vi "Mutation Frame.vi"(8 "error in (no error)":errorcluster, 10 "OSSP_Problem":refnum<class "OSSP_Problem.lvclass">, 11 "GA in":refnum<class "GA.lvclass">) -> (0 "error out":errorcluster, 2 "OSSP_Problem Out":refnum<class "OSSP_Problem.lvclass">, 3 "GA out":refnum<class "GA.lvclass">)   [LabVIEW 2013, in "GA.lvclass"]
uses:
  GA.lvclass
  OSSP_Problem.lvclass
  GA.lvclass/GA.ctl
  SA_Class/Controls/Perturbation Method.ctl
  OSSP_Problem.lvclass/OSSP_Problem.ctl
  SA.lvclass/SA.ctl
  SA_Class/Setters/Write Alpha Value.vi
  SA_Class/Setters/Write Current Temperature.vi
  SA_Class/Setters/Write Cooling Strategy.vi
  SA_Class/Setters/Write Initial Temperature.vi
  SA_Class/Setters/Write Stop Temperature.vi
  SA_Class/Setters/Write Cooling Rate.vi
  SA_Class/Setters/Write Epoch Length.vi
  SA_Class/Setters/Write Current Solution.vi
  SA_Class/Setters/Write Best Solution.vi
  GA/SubVIS/Calcualte General Tardiness.vi
  Scheduler_Class/Giffler Thompson Active Schedule Engine.vi
  Scheduler_Class/MyFIFOScheduler.vi
  Scheduler_Class/Calculate Makespan.vi
  Scheduler_Class/Job Completion Times.vi
  Scheduler_Class/Reorder Chromosome  After Makespan Calculation.vi
  Scheduler_Class/Prins FIFO Scheduler Methods and Controls/Methods/Calculate Final Completion Times of Jobs.vi
  Scheduler_Class/Prins FIFO Scheduler Methods and Controls/Methods/Reorder Schedule(Prins FIFO) based on Start Times.vi
  Scheduler_Class/Prins FIFO Scheduler Methods and Controls/Prins FIFO Scheduler.vi
  SA_Class/Perturb Current Solution.vi
  SA_Class/Getters/Read Current Solution.vi
  SA_Class/Setters/Write New Solution.vi
  SA_Class/Getters/Read New Solution.vi
  SA_Class/Calculate Acceptance Probability.vi
  SA_Class/Getters/Read Best Solution.vi
  SA_Class/Getters/Read Epoch Length.vi
  SA_Class/Getters/Read Current Temperature.vi
  SA_Class/Getters/Read Cooling Strategy.vi
  SA_Class/Getters/Read Cooling Rate.vi
  SA_Class/Getters/Read Alpha Value.vi
  SA_Class/Getters/Read Stop Temperature.vi
  Getters/Read Scheduler.vi
  Getters/Read Objective .vi
  Getters/Read Reorder.vi
  Scheduler_Class/Operation to Machine Job Tuple.vi
  Scheduler_Class/Check Other Machines for Schedule Time.vi
  Scheduler_Class/Schedule Job.vi
  Scheduler_Class/Find Gaps on Particular Machine.vi
  Scheduler_Class/Increment Number of Jobs on Machine.vi
  Scheduler_Class/Find Job On Other Machines.vi
  Scheduler_Class/Prins FIFO Scheduler Methods and Controls/Methods/UpdateMachineGaps.vi
  Scheduler_Class/Prins FIFO Scheduler Methods and Controls/Methods/UpdateJobGaps.vi
  Scheduler_Class/Prins FIFO Scheduler Methods and Controls/Methods/Find Intersecting Gaps.vi
  <vilib>/Analysis/1siggen.llb/Riffle Array (I32).vi
  Scheduler_Class/GT Algorithm Find M_ok and J_ok.vi
  Scheduler_Class/Prins FIFO Scheduler Methods and Controls/Methods/Transform to Plain Job and Machine Gaps Array.vi
  SA.lvclass
  <vilib>/Analysis/NI_AALBase.lvlib
  Scheduler.lvclass
panel:
  out "SPT":u16[](array[numeric])
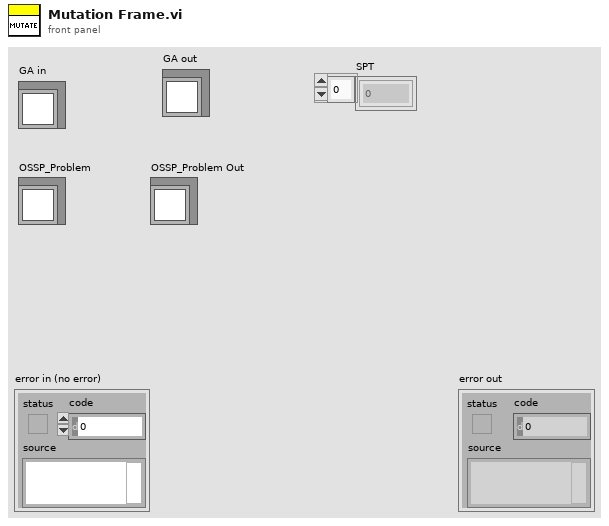
[diagram p1: front panel]
types:
  T1 = typedef "SA.lvclass/Perturbation Method.ctl" = enum16{"Simple Swap", "Insert", "NonRedundantSwap", "Job Order Swap", "Machine Order Swap", "Machine&Job Order Swap", "Critical Path Swap"}
  T2 = typedef "Solution_GA.ctl" = cluster{"Schedule":u16[], "Fitness":u16, "Fitness Valid?":bool}
  T3 = typedef "GA.lvclass/Mutation Type.ctl" = enum16{"Swap", "Non-Redundant Swap", "Insert", "Shift", "Shuflle", "Inversion", "SA", "IRH3T", "JO4M Swap", "MO4J Swap", "SPT JO4M", "SPT MO4J", "LCTJ Swap", "Low's Mutation", "ND Mutation"}
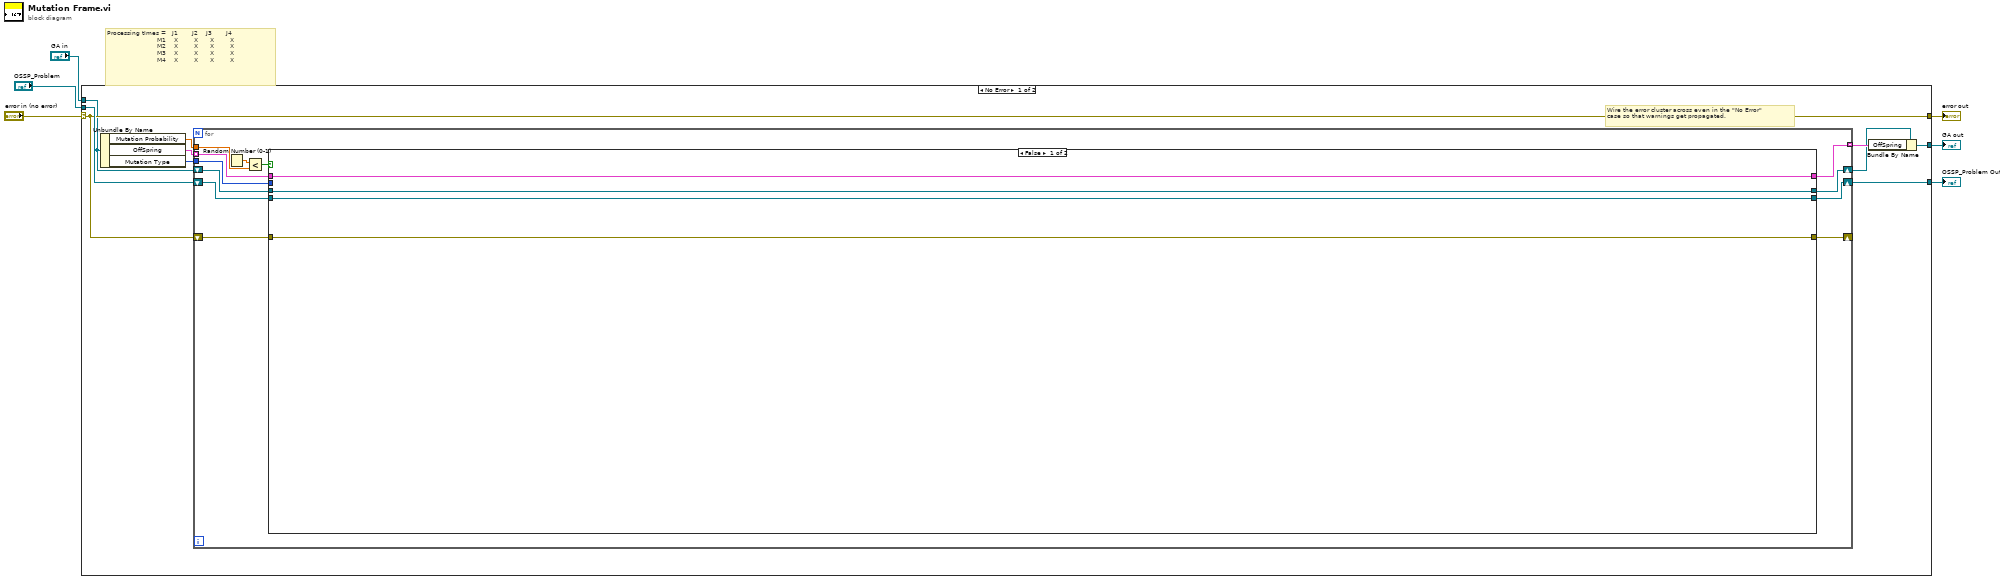
[diagram p0: block diagram]
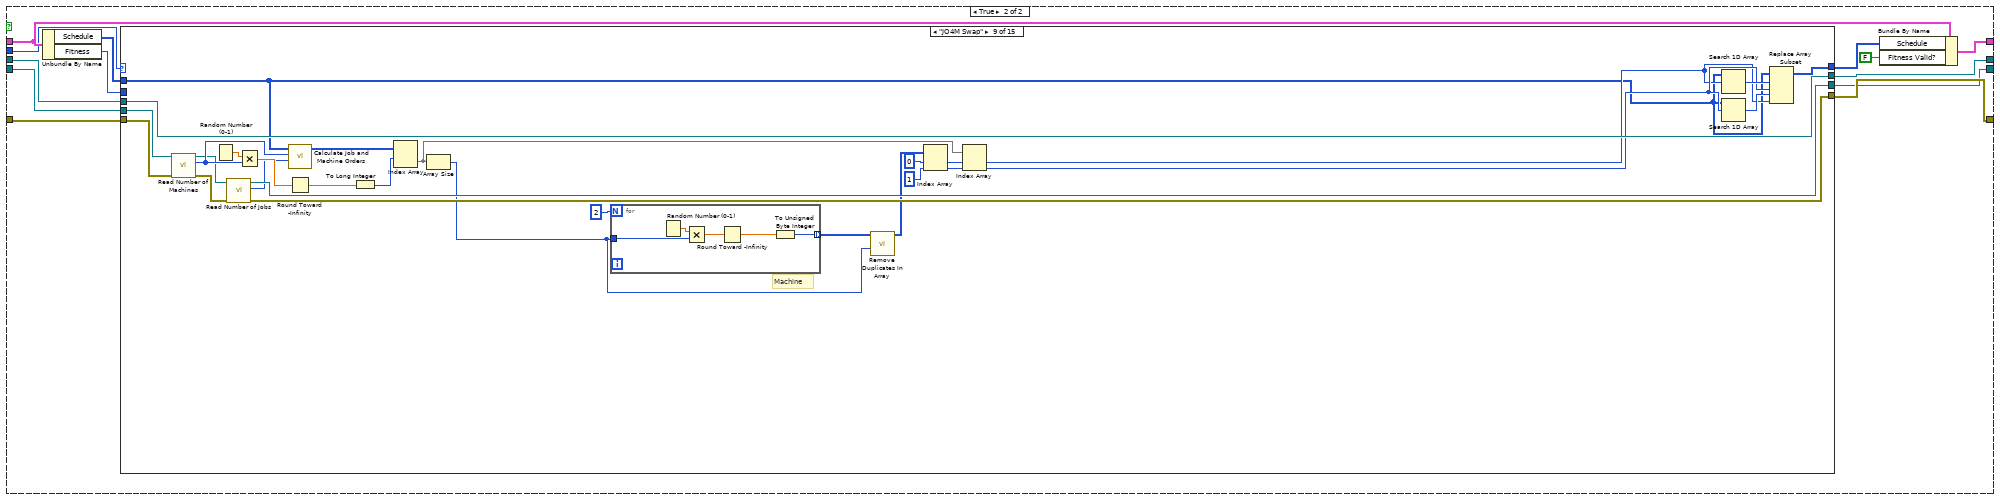
[diagram p2: hidden frame]
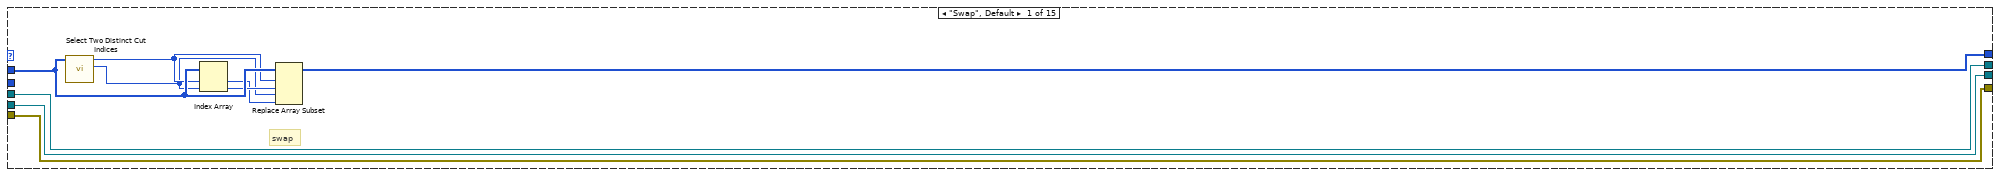
[diagram p3: hidden frame]
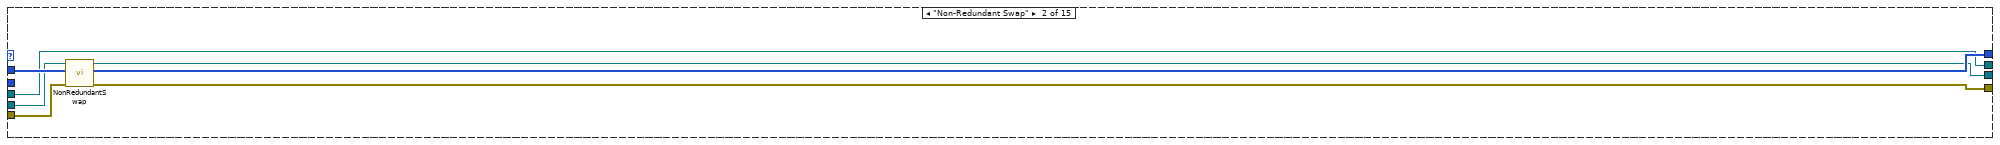
[diagram p4: hidden frame]
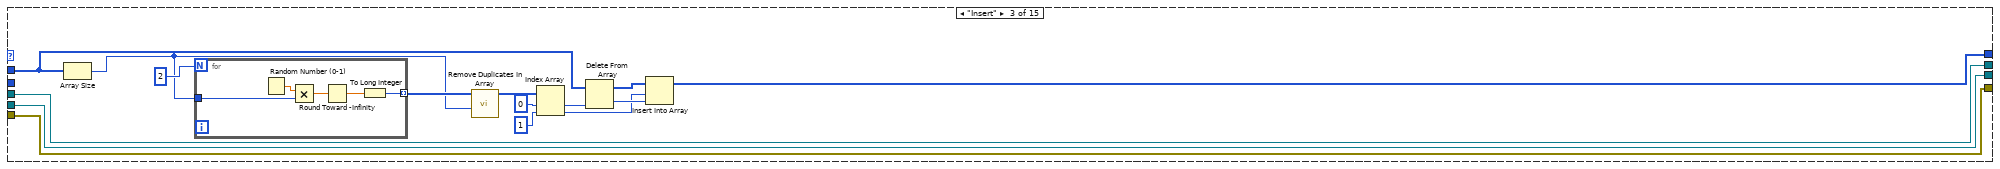
[diagram p5: hidden frame]
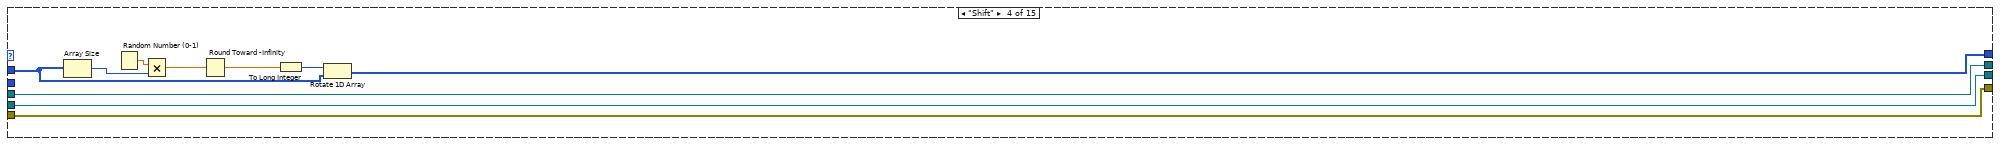
[diagram p6: hidden frame]
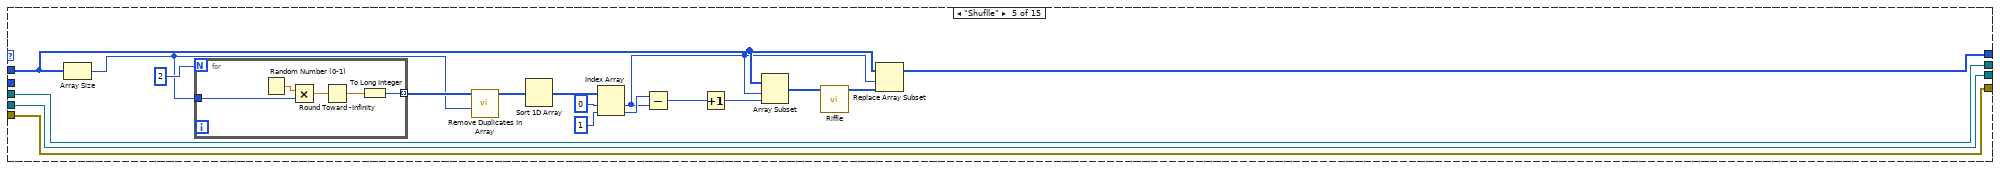
[diagram p7: hidden frame]
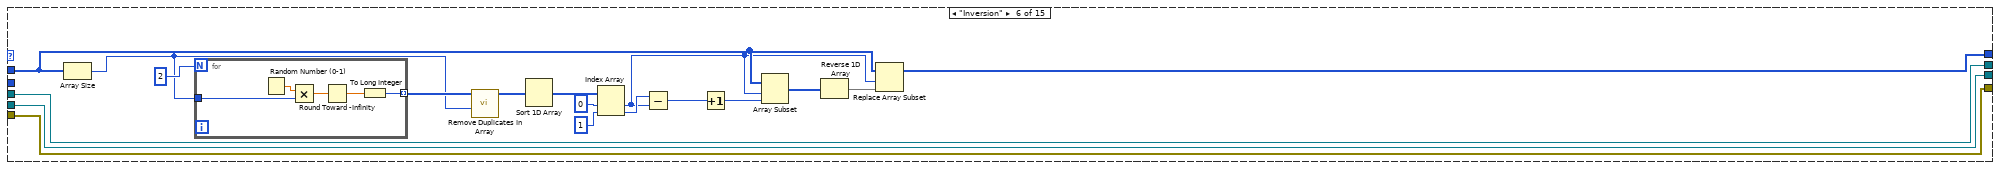
[diagram p8: hidden frame]
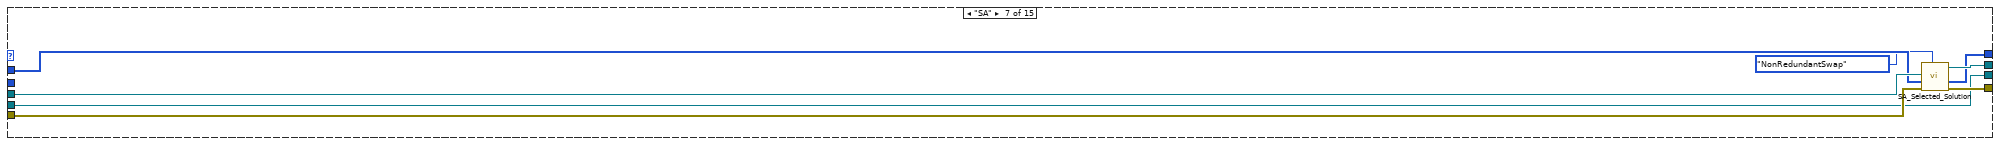
[diagram p9: hidden frame]
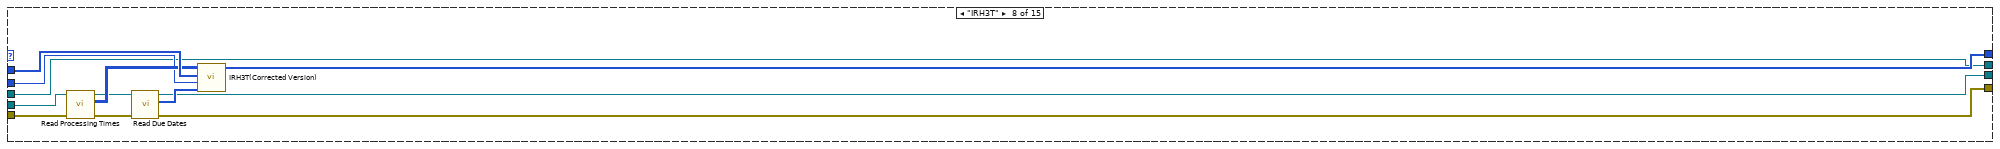
[diagram p10: hidden frame]
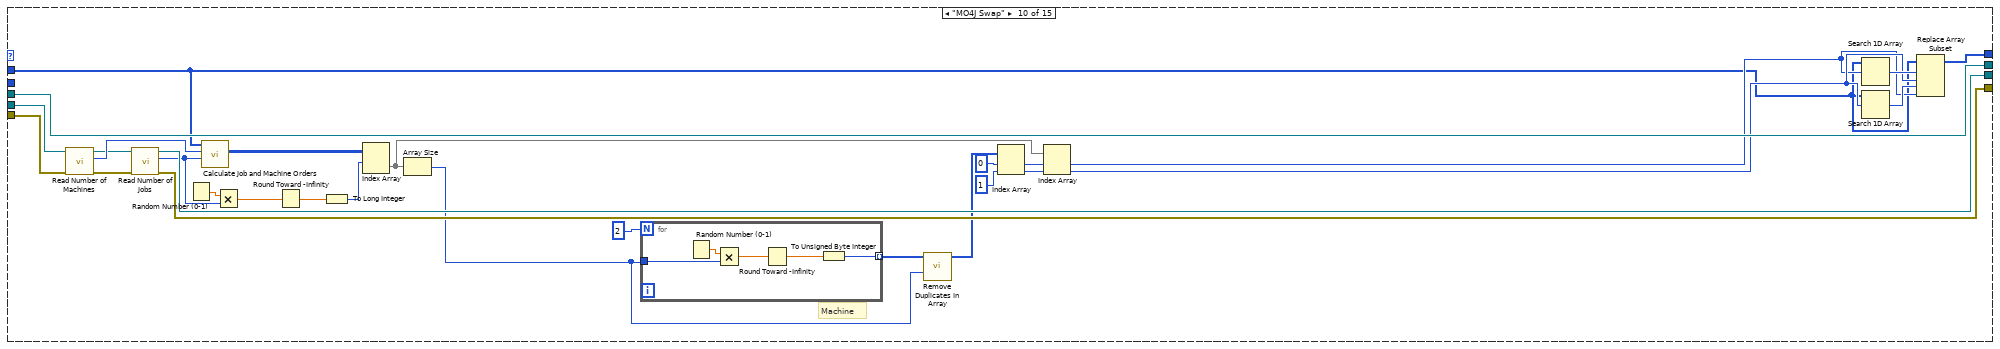
[diagram p11: hidden frame]
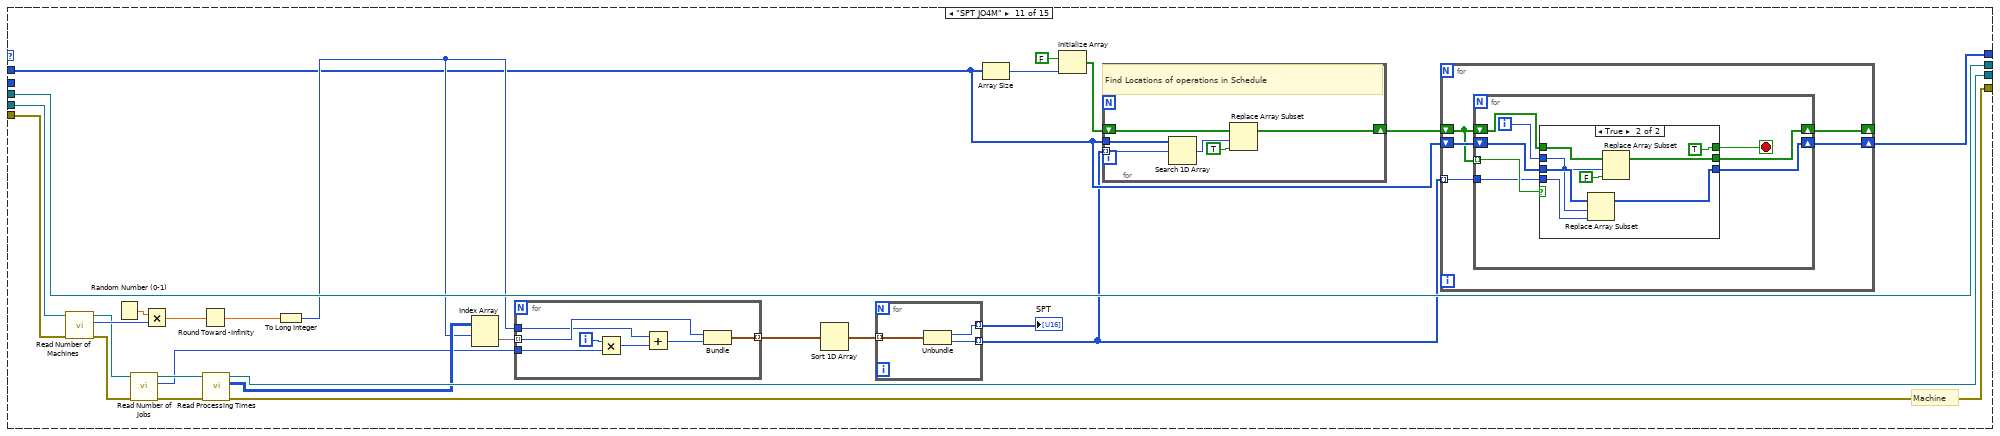
[diagram p12: hidden frame]
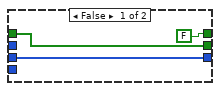
[diagram p13: hidden frame]
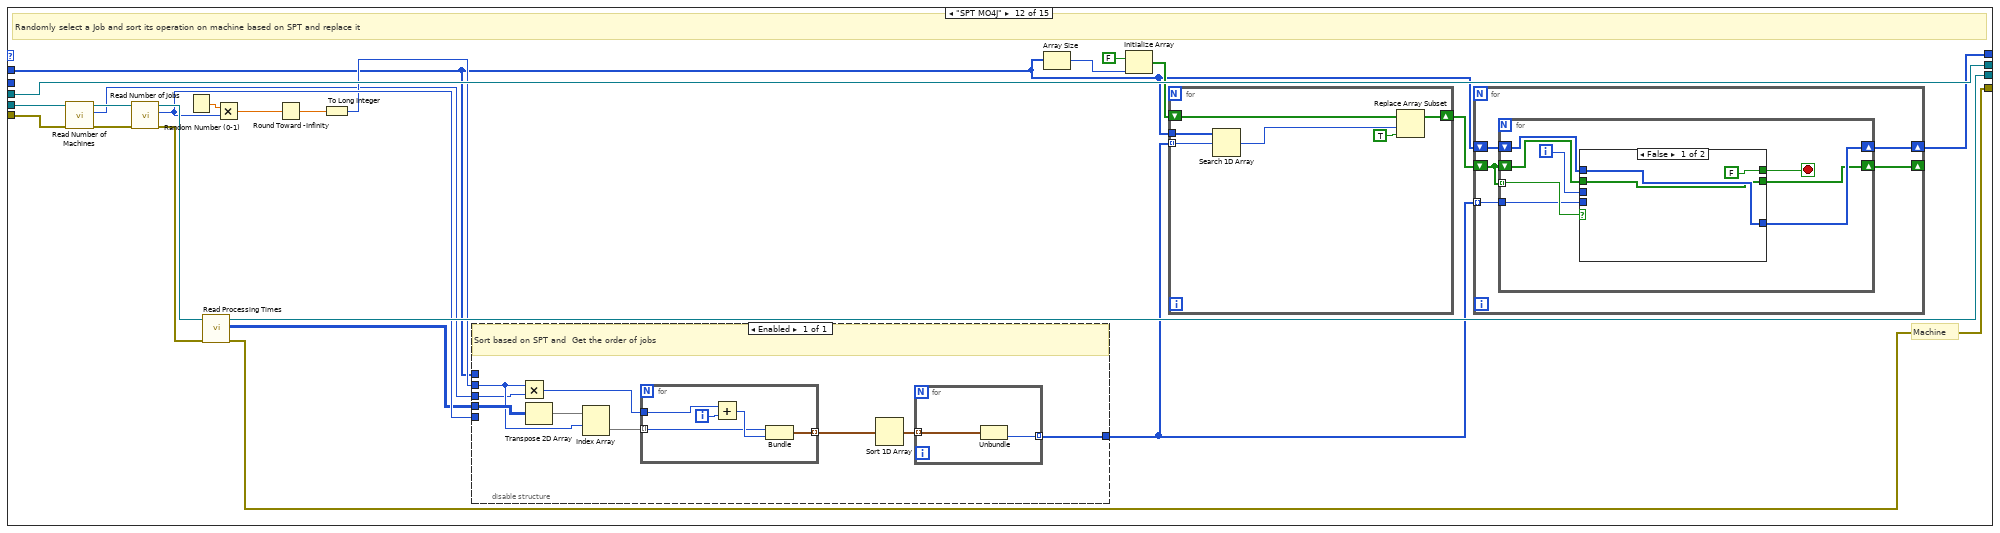
[diagram p14: hidden frame]
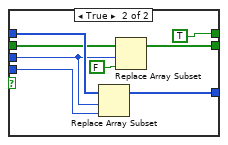
[diagram p15: hidden frame]
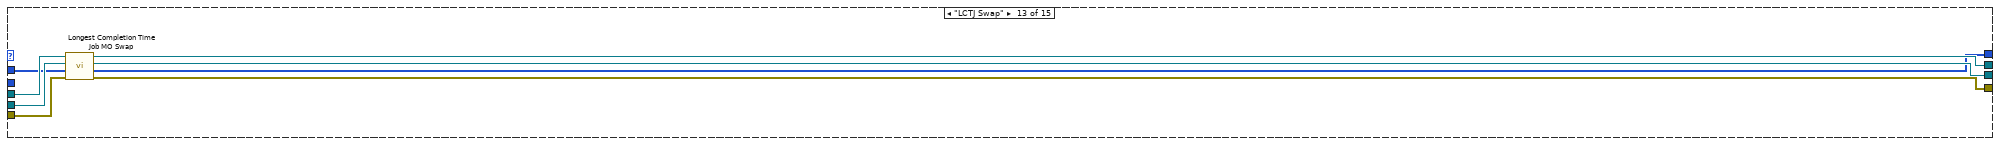
[diagram p16: hidden frame]
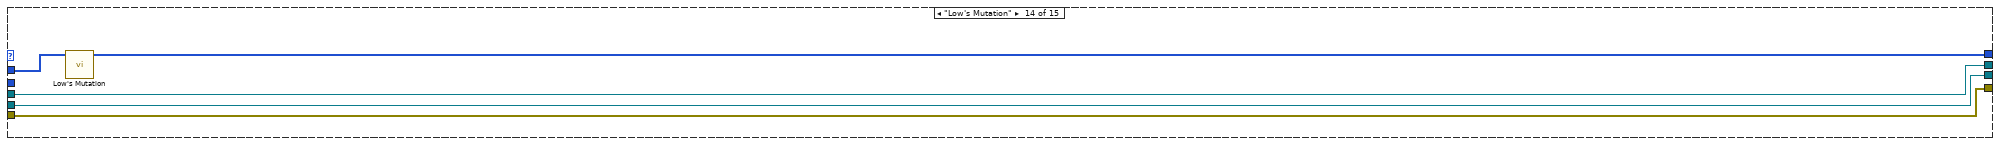
[diagram p17: hidden frame]
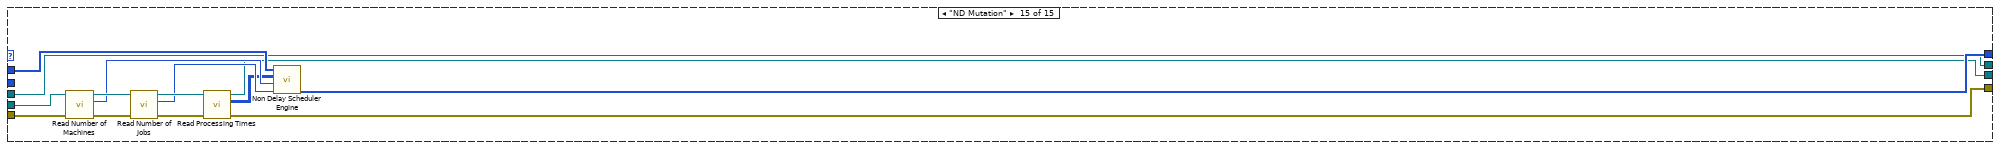
[diagram p18: hidden frame]
diagram:
  # "Processing tImes =   J1       J2    J3       J4   \n                         M1    X        X      X        X\n                         M2    X        X      X        X\n                         M3    X        X      X        X\n                         M4    X        X      X        X"
  n1 = case shown="No Error" "error in (no error)" {
    selector: "error in (no error)" -> [w9 w391]
    tunnel: [w9 w391] -> w5
    tunnel: [w13 w390] -> w3
    tunnel: "GA in" -> [w8 w390]
    tunnel: "OSSP_Problem" -> [w10 w389]
    tunnel: [w11 w389] -> w1
    frame No Error {
      # "Wire the error cluster across even in the \"No Error\"\ncase so that warnings get propagated."
      n2 = Unbundle By Name(w8) -> ("Mutation Probability"=w15:dbl, "OffSpring"=w16:T2[], "Mutation Type"=w12:T3)
      n3 = for {
        tunnel: w16 -> [w26] mode=indexing
        tunnel: w15 -> [w27]
        tunnel: [w24] -> w14 mode=indexing
        tunnel: w12 -> [w23]
        shift-right: [w17] -> w11
        shift-left: w10 -> [w18]
        shift-right: [w21] -> _
        shift-left: w9 -> [w22]
        shift-right: [w19] -> w7
        shift-left: w8 -> [w20]
        n4 = Random Number (0-1)() -> (number: 0 to 1=w28:dbl)
        n5 = Less?(x=w28, y=w27) -> (x < y?=w25:bool)
        n6 = case shown="False" w25 {
          tunnel: w26 -> [w32 w44]
          tunnel: [w32 w41] -> w24
          tunnel: w23 -> [_ w40]
          tunnel: w22 -> [w31 w39]
          tunnel: [w31 w38] -> w21
          tunnel: w20 -> [w30 w37]
          tunnel: [w30 w36] -> w19
          tunnel: w18 -> [w29 w34]
          tunnel: [w29 w33] -> w17
          frame False {
          }
          frame True {
            n7 = Unbundle By Name(w44) -> ("Schedule"=w45:u16[], "Fitness"=w35:u16)
            n8 = case shown="\"JO4M Swap\"" w40 {
              tunnel: w45 -> [w54 w61 w76 w88 w109 w132 w142 w157 w163 w198 w230 w294 w363 w371 w388]
              tunnel: [w53 w58 w74 w85 w108 w131 w143 w150 w172 w206 w227 w298 w362 w370 w378] -> w43
              tunnel: w39 -> [w48 w60 w64 w84 w94 w130 w141 w152 w171 w205 w248 w311 w367 w374 w380]
              tunnel: [w48 w59 w64 w84 w94 w130 w140 w147 w165 w199 w240 w304 w366 w374 w379] -> w38
              tunnel: w37 -> [w47 w57 w63 w83 w93 w129 w145 w148 w186 w220 w252 w315 w369 w373 w377]
              tunnel: [w47 w57 w63 w83 w93 w129 w144 w148 w186 w220 w252 w315 w368 w373 w377] -> w36
              tunnel: w35 -> [_ _ _ _ _ _ _ w155 _ _ _ _ _ _ _]
              tunnel: w34 -> [w46 w56 w62 w82 w92 w128 w139 w149 w170 w204 w247 w310 w365 w372 w376]
              tunnel: [w46 w55 w62 w82 w92 w128 w139 w146 w167 w201 w242 w306 w364 w372 w375] -> w33
              frame "Swap", Default {
                # "swap"
                n9 = call "Select Two Distinct Cut Indices.vi"("Schedule"=w54) -> ("Index 2"=w49:i32, "Index 1"=w50:i32)  [unwired: 9 in]
                n10 = Index Array(array=w54, index #1=w50, index #2=w49) -> (element #1=w51:u16, element #2=w52:u16)
                n11 = Replace Array Subset(array=w54, new element #1=w52, index #1=w50, new element #2=w51, index #2=w49) -> (w53:u16[])
              }
              frame "Non-Redundant Swap" {
                n12 = call "NonRedundantSwap.vi"("error in (no error)"=w60, "Schedule in"=w61, "OSSP_Problem in"=w56) -> ("error out"=w59:errorcluster, "Schedule out"=w58:u16[], "OSSP_Problem out"=w55:refnum<class "OSSP_Problem.lvclass">)  [unwired: 6 in]
              }
              frame "Insert" {
                n13 = Array Size(array=w76) -> (size(s)=w68:i32)
                n14 = for {
                  N: 2 -> [_]
                  tunnel: w68 -> [w78]
                  tunnel: [w77] -> w69 mode=indexing
                  n15 = Random Number (0-1)() -> (number: 0 to 1=w81:dbl)
                  n16 = Multiply(x=w81, y=w78) -> (x*y=w80:dbl)
                  n17 = Round Toward -Infinity(1:w80) -> (0:w79:dbl)
                  n18 = To Long Integer(number=w79) -> (32bit integer=w77:i32)
                }
                n19 = call "Remove Duplicates In Array.vi"("Max Index Bound"=w68, "Random Numbers Array"=w69) -> ("Random Numbers Array without Duplicates"=w67:i32[])  [unwired: 9 in]
                n20 = Index Array(array=w67, index #1=0 ("index"), index #2=1 ("index")) -> (element #1=w73:i32, element #2=w71:i32)
                n21 = Delete From Array(array=w76, index=w73) -> (deleted portion=w72:u16, array with subset deleted=w75:u16[])  [unwired: 1 in]
                n22 = Insert Into Array(array=w75, index=w71, new element=w72) -> (w74:u16[])
              }
              frame "Shift" {
                n23 = Array Size(array=w88) -> (size(s)=w90:i32)
                n24 = Random Number (0-1)() -> (number: 0 to 1=w91:dbl)
                n25 = Multiply(x=w91, y=w90) -> (x*y=w89:dbl)
                n26 = Round Toward -Infinity(1:w89) -> (0:w87:dbl)
                n27 = To Long Integer(number=w87) -> (32bit integer=w86:i32)
                n28 = Rotate 1D Array(1:w88, 2:w86) -> (0:w85:u16[])
              }
              frame "Shuflle" {
                n29 = Array Size(array=w109) -> (size(s)=w105:i32)
                n30 = for {
                  N: 2 -> [_]
                  tunnel: w105 -> [w111]
                  tunnel: [w110] -> w106 mode=indexing
                  n31 = Random Number (0-1)() -> (number: 0 to 1=w114:dbl)
                  n32 = Multiply(x=w114, y=w111) -> (x*y=w113:dbl)
                  n33 = Round Toward -Infinity(1:w113) -> (0:w112:dbl)
                  n34 = To Long Integer(number=w112) -> (32bit integer=w110:i32)
                }
                n35 = call "Remove Duplicates In Array.vi"("Max Index Bound"=w105, "Random Numbers Array"=w106) -> ("Random Numbers Array without Duplicates"=w102:i32[])  [unwired: 9 in]
                n36 = Sort 1D Array(array=w102) -> (sorted array=w101:i32[])
                n37 = Index Array(array=w101, index #1=0 ("index"), index #2=1 ("index")) -> (element #1=w98:i32, element #2=w100:i32)
                n38 = Subtract(x=w100, y=w98) -> (x-y=w96:i32)
                n39 = Increment(x=w96) -> (x+1=w95:i32)
                n40 = Array Subset(array=w109, index=w98, length=w95) -> (w99:u16[])
                n41 = call-poly <vilib>:"Riffle.vi"("X"=w99) -> ("Riffled {X}"=w97:i32[])  [unwired: 8 in, 2 out]
                n42 = Replace Array Subset(array=w109, new element=w97, index=w98) -> (w108:u16[])
              }
              frame "Inversion" {
                n43 = Array Size(array=w132) -> (size(s)=w125:i32)
                n44 = for {
                  N: 2 -> [_]
                  tunnel: w125 -> [w134]
                  tunnel: [w133] -> w126 mode=indexing
                  n45 = Random Number (0-1)() -> (number: 0 to 1=w137:dbl)
                  n46 = Multiply(x=w137, y=w134) -> (x*y=w136:dbl)
                  n47 = Round Toward -Infinity(1:w136) -> (0:w135:dbl)
                  n48 = To Long Integer(number=w135) -> (32bit integer=w133:i32)
                }
                n49 = call "Remove Duplicates In Array.vi"("Max Index Bound"=w125, "Random Numbers Array"=w126) -> ("Random Numbers Array without Duplicates"=w122:i32[])  [unwired: 9 in]
                n50 = Sort 1D Array(array=w122) -> (sorted array=w121:i32[])
                n51 = Index Array(array=w121, index #1=0 ("index"), index #2=1 ("index")) -> (element #1=w119:i32, element #2=w120:i32)
                n52 = Subtract(x=w120, y=w119) -> (x-y=w116:i32)
                n53 = Increment(x=w116) -> (x+1=w115:i32)
                n54 = Array Subset(array=w132, index=w119, length=w115) -> (w118:u16[])
                n55 = Reverse 1D Array(array=w118) -> (reversed array=w117:u16[])
                n56 = Replace Array Subset(array=w132, new element=w117, index=w119) -> (w131:u16[])
              }
              frame "SA" {
                n57 = call "SA_Selected_Solution.vi"("Perturbation Method"=Perturbation_Method."NonRedundantSwap", "error in (no error)"=w141, "Schedule In"=w142, "GA.lvclass"=w145) -> ("error out"=w140:errorcluster, "Schedule Out"=w143:u16[], "GA out"=w144:refnum<class "GA.lvclass">)  [unwired: 3 in, 2 out]
              }
              frame "IRH3T" {
                n58 = call "Read Processing Times.vi"("error in (no error)"=w152, "OSSP_Problem in"=w149) -> ("error out"=w153:errorcluster, "Processing Times"=w156:u16[][], "OSSP_Problem out"=w154:refnum<class "OSSP_Problem.lvclass">)  [unwired: 7 in]
                n59 = call "Read Due Dates.vi"("error in (no error)"=w153, "OSSP_Problem in"=w154) -> ("error out"=w147:errorcluster, "Due Dates"=w151:u16[], "OSSP_Problem out"=w146:refnum<class "OSSP_Problem.lvclass">)  [unwired: 7 in]
                n60 = call "IRH3T(Corrected Version).vi"("Due Dates"=w151, "Initial Tardiness"=w155, "Schedule 2B Improved"=w157, "Proocessing Times  (Machines x Jobs)"=w156) -> ("IRH3T (Reordered) Schedule Out"=w150:u16[])  [unwired: 5 in, 2 out]
              }
              frame "JO4M Swap" {
                # "Machine"
                n61 = call "Read Number of Machines.vi"("error in (no error)"=w171, "OSSP_Problem in"=w170) -> ("error out"=w166:errorcluster, "Number of Machines"=w169:i32, "OSSP_Problem out"=w168:refnum<class "OSSP_Problem.lvclass">)  [unwired: 7 in]
                n62 = Random Number (0-1)() -> (number: 0 to 1=w185:dbl)
                n63 = call "Read Number of Jobs.vi"("error in (no error)"=w166, "OSSP_Problem in"=w168) -> ("error out"=w165:errorcluster, "Number of Jobs"=w164:i32, "OSSP_Problem out"=w167:refnum<class "OSSP_Problem.lvclass">)  [unwired: 7 in]
                n64 = Multiply(x=w185, y=w169) -> (x*y=w184:dbl)
                n65 = call "Calculate Job and Machine Orders.vi"("Number of Jobs"=w164, "Number of Machines"=w169, "Schedule"=w163) -> ("JO4M"=w158:u16[][])  [unwired: 7 in, 1 out]
                n66 = Round Toward -Infinity(1:w184) -> (0:w183:dbl)
                n67 = To Long Integer(number=w183) -> (32bit integer=w178:i32)
                n68 = Index Array(array=w158, index (row)=w178) -> (element=w177:u16[])  [unwired: 1 in]
                n69 = Array Size(array=w177) -> (size(s)=w159:i32)
                n70 = for {
                  N: 2 -> [_]
                  tunnel: w159 -> [w190]
                  tunnel: [w187] -> w162 mode=indexing
                  n71 = Random Number (0-1)() -> (number: 0 to 1=w191:dbl)
                  n72 = Multiply(x=w191, y=w190) -> (x*y=w189:dbl)
                  n73 = Round Toward -Infinity(1:w189) -> (0:w188:dbl)
                  n74 = To Unsigned Byte Integer(number=w188) -> (unsigned 8bit integer=w187:u8)
                }
                n75 = call "Remove Duplicates In Array.vi"("Max Index Bound"=w159, "Random Numbers Array"=w162) -> ("Random Numbers Array without Duplicates"=w160:i32[])  [unwired: 9 in]
                n76 = Index Array(array=w160, index #1=0 ("index"), index #2=1 ("index")) -> (element #1=w180:i32, element #2=w179:i32)
                n77 = Index Array(array=w177, index #1=w180, index #2=w179) -> (element #1=w173:u16, element #2=w175:u16)
                n78 = Search 1D Array(1D array=w163, element=w173) -> (index of element=w176:i32)  [unwired: 1 in]
                n79 = Search 1D Array(1D array=w163, element=w175) -> (index of element=w174:i32)  [unwired: 1 in]
                n80 = Replace Array Subset(array=w163, new element #1=w175, index #1=w176, new element #2=w173, index #2=w174) -> (w172:u16[])
              }
              frame "MO4J Swap" {
                # "Machine"
                n81 = call "Read Number of Machines.vi"("error in (no error)"=w205, "OSSP_Problem in"=w204) -> ("error out"=w200:errorcluster, "Number of Machines"=w203:i32, "OSSP_Problem out"=w202:refnum<class "OSSP_Problem.lvclass">)  [unwired: 7 in]
                n82 = call "Read Number of Jobs.vi"("error in (no error)"=w200, "OSSP_Problem in"=w202) -> ("error out"=w199:errorcluster, "Number of Jobs"=w192:i32, "OSSP_Problem out"=w201:refnum<class "OSSP_Problem.lvclass">)  [unwired: 7 in]
                n83 = Random Number (0-1)() -> (number: 0 to 1=w219:dbl)
                n84 = call "Calculate Job and Machine Orders.vi"("Number of Jobs"=w192, "Number of Machines"=w203, "Schedule"=w198) -> ("MO4J"=w193:u16[][])  [unwired: 7 in, 1 out]
                n85 = Multiply(x=w219, y=w192) -> (x*y=w218:dbl)
                n86 = Round Toward -Infinity(1:w218) -> (0:w217:dbl)
                n87 = To Long Integer(number=w217) -> (32bit integer=w212:i32)
                n88 = Index Array(array=w193, index (row)=w212) -> (element=w211:u16[])  [unwired: 1 in]
                n89 = Array Size(array=w211) -> (size(s)=w194:i32)
                n90 = for {
                  N: 2 -> [_]
                  tunnel: w194 -> [w224]
                  tunnel: [w221] -> w197 mode=indexing
                  n91 = Random Number (0-1)() -> (number: 0 to 1=w225:dbl)
                  n92 = Multiply(x=w225, y=w224) -> (x*y=w223:dbl)
                  n93 = Round Toward -Infinity(1:w223) -> (0:w222:dbl)
                  n94 = To Unsigned Byte Integer(number=w222) -> (unsigned 8bit integer=w221:u8)
                }
                n95 = call "Remove Duplicates In Array.vi"("Max Index Bound"=w194, "Random Numbers Array"=w197) -> ("Random Numbers Array without Duplicates"=w195:i32[])  [unwired: 9 in]
                n96 = Index Array(array=w195, index #1=0 ("index"), index #2=1 ("index")) -> (element #1=w214:i32, element #2=w213:i32)
                n97 = Index Array(array=w211, index #1=w214, index #2=w213) -> (element #1=w207:u16, element #2=w209:u16)
                n98 = Search 1D Array(1D array=w198, element=w207) -> (index of element=w210:i32)  [unwired: 1 in]
                n99 = Search 1D Array(1D array=w198, element=w209) -> (index of element=w208:i32)  [unwired: 1 in]
                n100 = Replace Array Subset(array=w198, new element #1=w209, index #1=w210, new element #2=w207, index #2=w208) -> (w206:u16[])
              }
              frame "SPT JO4M" {
                # "Machine"
                n101 = call "Read Number of Machines.vi"("error in (no error)"=w248, "OSSP_Problem in"=w247) -> ("error out"=w244:errorcluster, "Number of Machines"=w246:i32, "OSSP_Problem out"=w245:refnum<class "OSSP_Problem.lvclass">)  [unwired: 7 in]
                n102 = Random Number (0-1)() -> (number: 0 to 1=w251:dbl)
                n103 = call "Read Number of Jobs.vi"("error in (no error)"=w244, "OSSP_Problem in"=w245) -> ("error out"=w241:errorcluster, "Number of Jobs"=w237:i32, "OSSP_Problem out"=w243:refnum<class "OSSP_Problem.lvclass">)  [unwired: 7 in]
                n104 = Multiply(x=w251, y=w246) -> (x*y=w250:dbl)
                n105 = Round Toward -Infinity(1:w250) -> (0:w249:dbl)
                n106 = call "Read Processing Times.vi"("error in (no error)"=w241, "OSSP_Problem in"=w243) -> ("error out"=w240:errorcluster, "Processing Times"=w239:u16[][], "OSSP_Problem out"=w242:refnum<class "OSSP_Problem.lvclass">)  [unwired: 7 in]
                n107 = To Long Integer(number=w249) -> (32bit integer=w236:i32)
                n108 = Index Array(array=w239, index (row)=w236) -> (element=w238:u16[])  [unwired: 1 in]
                n109 = for {
                  tunnel: w238 -> [w292] mode=indexing
                  tunnel: w237 -> [w291]
                  tunnel: w236 -> [w289]
                  tunnel: [w286] -> w235 mode=indexing
                  i -> [w290]
                  n110 = Multiply(x=w290, y=w291) -> (x*y=w288:i32)
                  n111 = Add(x=w289, y=w288) -> (x+y=w287:i32)
                  n112 = Bundle("Numeric"=w292, w287) -> (w286:cluster{"Numeric":u16, i32})  [unwired: 1 in]
                }
                n113 = Sort 1D Array(array=w235) -> (sorted array=w234:cluster{"Numeric":u16, i32}[])
                n114 = for {
                  tunnel: w234 -> [w285] mode=indexing
                  tunnel: [w284] -> w228 mode=indexing
                  tunnel: [w283] -> w226 mode=indexing
                  n115 = Unbundle(w285) -> ("Numeric"=w283:u16, w284:i32)
                }
                "SPT" <- w226
                n116 = Array Size(array=w230) -> (size(s)=w232:i32)
                n117 = Initialize Array(FALSE, w232) -> (w231:bool[])
                n118 = for {
                  tunnel: w230 -> [w282]
                  tunnel: w228 -> [w281] mode=indexing
                  shift-right: [w277] -> w229
                  shift-left: w231 -> [w280]
                  # "Find Locations of operations in Schedule"
                  n119 = Search 1D Array(1D array=w282, element=w281) -> (index of element=w279:i32)  [unwired: 1 in]
                  n120 = Replace Array Subset(array=w280, new element=TRUE ("new element/subarray"), index=w279) -> (w277:bool[])
                }
                n121 = for {
                  shift-right: [w254] -> w227
                  shift-left: w230 -> [w257]
                  tunnel: w228 -> [w256] mode=indexing
                  shift-right: [w253] -> _
                  shift-left: w229 -> [w255]
                  n122 = for {
                    tunnel: w255 -> [w265] mode=indexing
                    shift-right: [w261] -> w254
                    shift-left: w257 -> [w264]
                    tunnel: w256 -> [w262]
                    shift-right: [w258] -> w253
                    shift-left: w255 -> [w259]
                    i -> [w263]
                    stop <- w260 stop-if-true
                    n123 = case shown="True" w265 {
                      tunnel: w264 -> [w268 w276]
                      tunnel: w263 -> [_ w271]
                      tunnel: w262 -> [_ w275]
                      tunnel: [w268 w273] -> w261
                      tunnel: [FALSE TRUE] -> w260
                      tunnel: w259 -> [w267 w272]
                      tunnel: [w267 w269] -> w258
                      frame False {
                      }
                      frame True {
                        n124 = Replace Array Subset(array=w276, new element=w275, index=w271) -> (w273:u16[])
                        n125 = Replace Array Subset(array=w272, new element=FALSE ("new element/subarray"), index=w271) -> (w269:bool[])
                      }
                    }
                  }
                }
              }
              frame "SPT MO4J" {
                # "Machine"
                # "Randomly select a Job and sort its operation on machine based on SPT and replace it"
                n126 = call "Read Number of Machines.vi"("error in (no error)"=w311, "OSSP_Problem in"=w310) -> ("error out"=w308:errorcluster, "Number of Machines"=w293:i32, "OSSP_Problem out"=w309:refnum<class "OSSP_Problem.lvclass">)  [unwired: 7 in]
                n127 = call "Read Number of Jobs.vi"("error in (no error)"=w308, "OSSP_Problem in"=w309) -> ("error out"=w305:errorcluster, "Number of Jobs"=w297:i32, "OSSP_Problem out"=w307:refnum<class "OSSP_Problem.lvclass">)  [unwired: 7 in]
                n128 = Random Number (0-1)() -> (number: 0 to 1=w314:dbl)
                n129 = call "Read Processing Times.vi"("error in (no error)"=w305, "OSSP_Problem in"=w307) -> ("error out"=w304:errorcluster, "Processing Times"=w296:u16[][], "OSSP_Problem out"=w306:refnum<class "OSSP_Problem.lvclass">)  [unwired: 7 in]
                n130 = Multiply(x=w314, y=w297) -> (x*y=w313:dbl)
                n131 = Round Toward -Infinity(1:w313) -> (0:w312:dbl)
                n132 = To Long Integer(number=w312) -> (32bit integer=w295:i32)
                n133 = disable-structure shown="Enabled" {
                  disable-tunnel: [w316] -> w299
                  disable-tunnel: w297 -> [_]
                  disable-tunnel: w296 -> [w324]
                  disable-tunnel: w295 -> [w321]
                  disable-tunnel: w294 -> [_]
                  disable-tunnel: w293 -> [w320]
                  frame Enabled {
                    # "Sort based on SPT and  Get the order of jobs"
                    n134 = Multiply(x=w321, y=w320) -> (x*y=w319:i32)
                    n135 = Transpose 2D Array(2D array=w324) -> (transposed array=w323:u16[][])
                    n136 = Index Array(array=w323, index (row)=w321) -> (element=w322:u16[])  [unwired: 1 in]
                    n137 = for {
                      tunnel: w322 -> [w328] mode=indexing
                      tunnel: w319 -> [w331]
                      tunnel: [w327] -> w318 mode=indexing
                      i -> [w330]
                      n138 = Add(x=w331, y=w330) -> (x+y=w329:i32)
                      n139 = Bundle("Numeric"=w328, w329) -> (w327:cluster{"Numeric":u16, i32})  [unwired: 1 in]
                    }
                    n140 = Sort 1D Array(array=w318) -> (sorted array=w317:cluster{"Numeric":u16, i32}[])
                    n141 = for {
                      tunnel: w317 -> [w326] mode=indexing
                      tunnel: [w325] -> w316 mode=indexing
                      n142 = Unbundle(w326) -> (w325:i32)  [unwired: 1 out]
                    }
                  }
                }
                n143 = Array Size(array=w294) -> (size(s)=w302:i32)
                n144 = Initialize Array(FALSE, w302) -> (w301:bool[])
                n145 = for {
                  tunnel: w294 -> [w361]
                  tunnel: w299 -> [w360] mode=indexing
                  shift-right: [w356] -> w300
                  shift-left: w301 -> [w359]
                  n146 = Search 1D Array(1D array=w361, element=w360) -> (index of element=w358:i32)  [unwired: 1 in]
                  n147 = Replace Array Subset(array=w359, new element=TRUE ("new element/subarray"), index=w358) -> (w356:bool[])
                }
                n148 = for {
                  shift-right: [w333] -> w298
                  shift-left: w294 -> [w336]
                  tunnel: w299 -> [w335] mode=indexing
                  shift-right: [w332] -> _
                  shift-left: w300 -> [w334]
                  n149 = for {
                    tunnel: w334 -> [w344] mode=indexing
                    shift-right: [w340] -> w333
                    shift-left: w336 -> [w343]
                    tunnel: w335 -> [w341]
                    shift-right: [w337] -> w332
                    shift-left: w334 -> [w338]
                    i -> [w342]
                    stop <- w339 stop-if-true
                    n150 = case shown="False" w344 {
                      tunnel: w343 -> [w347 w355]
                      tunnel: w342 -> [_ w350]
                      tunnel: w341 -> [_ w354]
                      tunnel: [w347 w352] -> w340
                      tunnel: [FALSE TRUE] -> w339
                      tunnel: w338 -> [w346 w351]
                      tunnel: [w346 w348] -> w337
                      frame False {
                      }
                      frame True {
                        n151 = Replace Array Subset(array=w355, new element=w354, index=w350) -> (w352:u16[])
                        n152 = Replace Array Subset(array=w351, new element=FALSE ("new element/subarray"), index=w350) -> (w348:bool[])
                      }
                    }
                  }
                }
              }
              frame "LCTJ Swap" {
                n153 = call "Longest Completion Time Job MO Swap.vi"("error in (no error)"=w367, "Schedule in"=w363, "OSSP_Problem"=w365, "GA in"=w369) -> ("error out"=w366:errorcluster, "Schedule out"=w362:u16[], "OSSP_Problem out"=w364:refnum<class "OSSP_Problem.lvclass">, "GA out"=w368:refnum<class "GA.lvclass">)  [unwired: 4 in]
              }
              frame "Low's Mutation" {
                n154 = call "Low's Mutation.vi"("Schedule"=w371) -> ("Mutated Solution"=w370:u16[])  [unwired: 10 in]
              }
              frame "ND Mutation" {
                n155 = call "Read Number of Machines.vi"("error in (no error)"=w380, "OSSP_Problem in"=w376) -> ("error out"=w387:errorcluster, "Number of Machines"=w383:i32, "OSSP_Problem out"=w385:refnum<class "OSSP_Problem.lvclass">)  [unwired: 7 in]
                n156 = call "Read Number of Jobs.vi"("error in (no error)"=w387, "OSSP_Problem in"=w385) -> ("error out"=w386:errorcluster, "Number of Jobs"=w382:i32, "OSSP_Problem out"=w384:refnum<class "OSSP_Problem.lvclass">)  [unwired: 7 in]
                n157 = call "Read Processing Times.vi"("error in (no error)"=w386, "OSSP_Problem in"=w384) -> ("error out"=w379:errorcluster, "Processing Times"=w381:u16[][], "OSSP_Problem out"=w375:refnum<class "OSSP_Problem.lvclass">)  [unwired: 7 in]
                n158 = call "Non Delay Scheduler Engine.vi"("Number of  Jobs"=w382, "Number of Machines"=w383, "Processing Times"=w381, "Schedule"=w388) -> ("Reordered Schedule"=w378:u16[])  [unwired: 2 in, 5 out]
              }
            }
            n159 = Bundle By Name(cluster=w44, "Schedule"=w43, "Fitness Valid?"=FALSE) -> (w41:T2)
          }
        }
      }
      n160 = Bundle By Name(cluster=w7, "OffSpring"=w14) -> (w13:refnum<class "GA.lvclass">)
    }
    frame Error {
    }
  }
  "error out" <- w5
  "GA out" <- w3
  "OSSP_Problem Out" <- w1
